vi "Convert BAR Pressure.vi"(1 "Input Byte 2":u8, 2 "Input Byte 1":u8) -> (0 "Pressure":dbl)   [LabVIEW 2011]
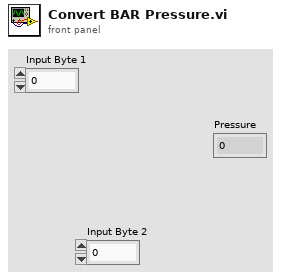
[diagram p1: front panel]
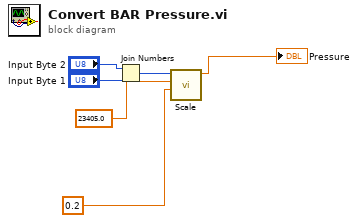
[diagram p0: block diagram]
diagram:
  n1 = Join Numbers(hi="Input Byte 2", lo="Input Byte 1") -> ((hi.lo)=w4:u16)
  n2 = call "Scale.vi"("Factor"=0.2, "FullScale"=23405.0, "Input"=w4) -> ("Output"=→"Pressure":dbl)  [unwired: 8 in]
